vi "IndividualOperations.vi"() -> ()   [LabVIEW 2021]
panel:
  in  "Slide":cluster{dbl, dbl}(slide)={0.0, 191.73664122137404} scale=0.0..255.0
  in  "U1":dbl(slide) scale=0.0..255.0
  in  "Enum 3":T1(ring)
  in  "Enum 2":enum16{"Rojo", "Verde", "Azul", "Color"}(ring)
  out "Waveform Graph 2":dbl[][](graph)
  out "Waveform Graph":dbl[][](graph)
  out "XY Graph":cluster{i32[], dbl[]}(graph)
  out "new picture":picture
  in  "Path":path
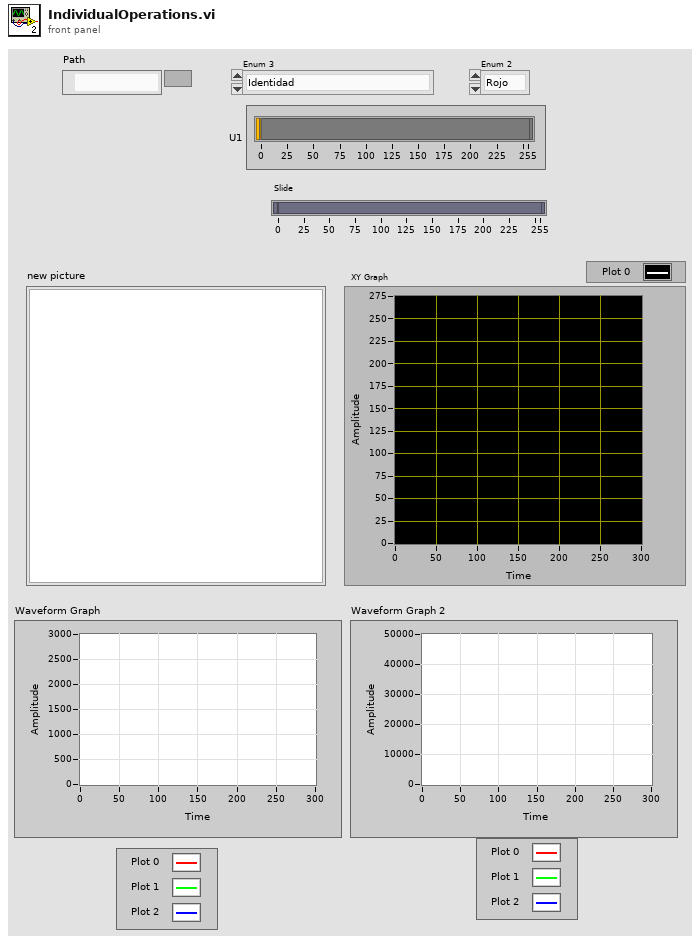
[diagram p1: front panel]
types:
  T1 = enum16{"Identidad", "Negativo", "Umbral", "Umbral Binario Por Intervalo", "Umbral Binario Por Intervalo Invertido", "Umbral Escala de Grises", "Extensión", "Reducción de nivel de grises"}
  T2 = typedef "imagedata.ctl" = cluster{"image type":i32, "image depth":i32, "image":u8[], "mask":u8[], "colors":u32[], "Rectangle":cluster{"left":i16, "top":i16, "right":i16, "bottom":i16}}
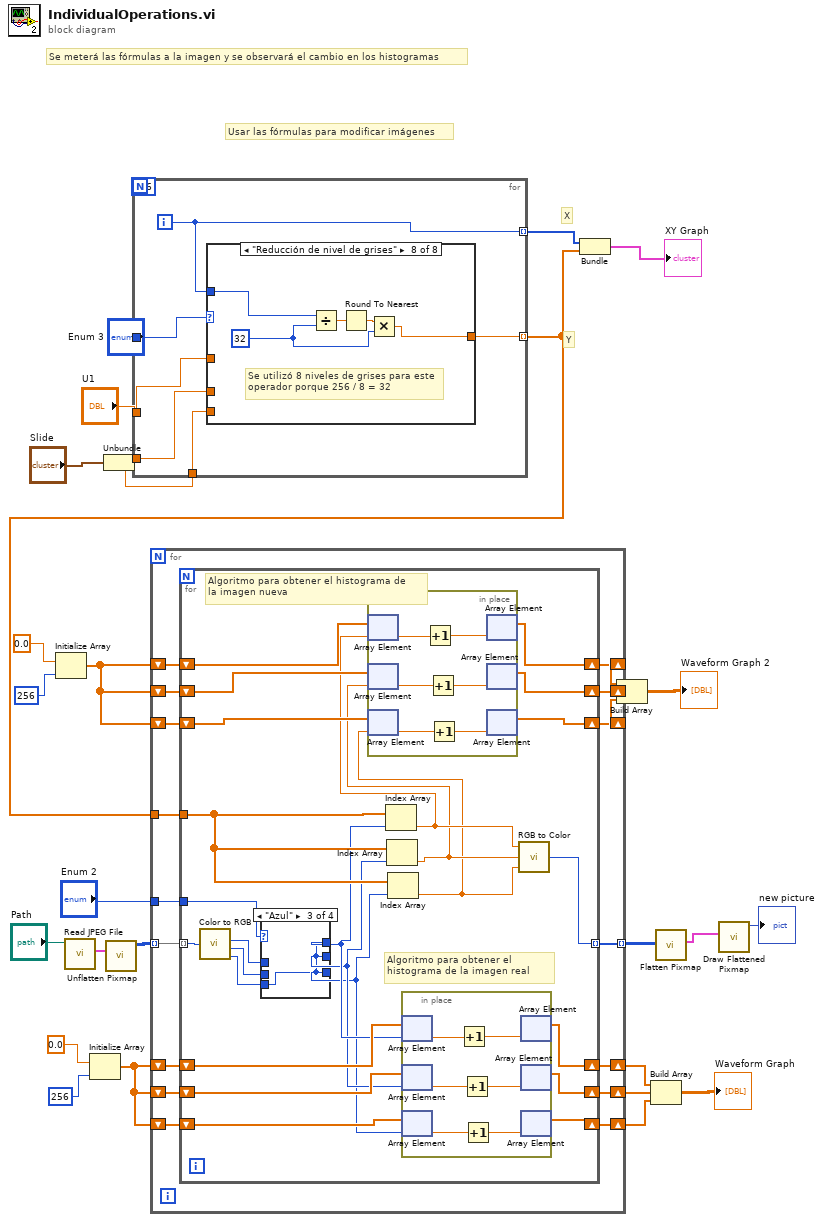
[diagram p0: block diagram]
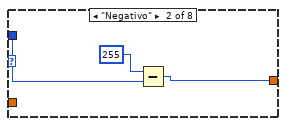
[diagram p3: hidden frame]
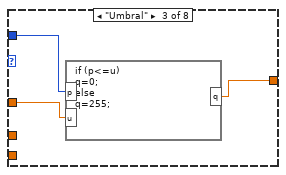
[diagram p4: hidden frame]
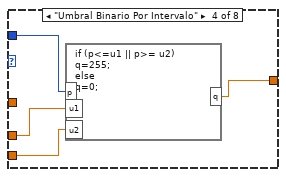
[diagram p5: hidden frame]
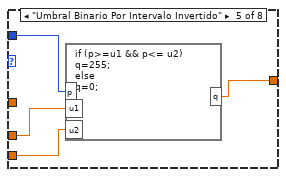
[diagram p6: hidden frame]
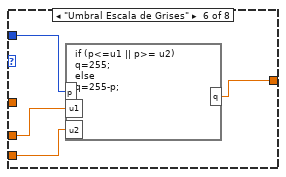
[diagram p7: hidden frame]
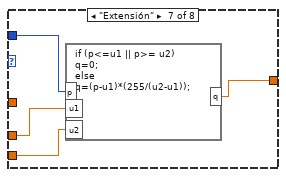
[diagram p8: hidden frame]
diagram:
  # "Usar las fórmulas para modificar imágenes"
  # "Se meterá las fórmulas a la imagen y se observará el cambio en los histogramas"
  # "Y"
  # "X"
  n1 = Initialize Array(0.0 ("element"), 256 ("dimension size")) -> (w9:dbl[])
  n2 = call <vilib>:"Read JPEG File.vi"("path to JPEG file"="Path") -> ("image data"=w29:T2)  [unwired: 8 in, 2 out]
  n3 = Initialize Array(0.0 ("element"), 256 ("dimension size")) -> (w19:dbl[])
  n4 = Unbundle("Slide") -> (w2:dbl, w1:dbl)
  n5 = call <vilib>:"Unflatten Pixmap.vi"("image data"=w29) -> ("24-bit pixmap"=w26:u32[][])  [unwired: 4 in, 6 out]
  n6 = for {
    N: 256 -> [_]
    tunnel: [w35] -> w23 mode=indexing
    tunnel: [w34] -> w14 mode=indexing
    tunnel: "Enum 3" -> [w36]
    tunnel: "U1" -> [w33]
    tunnel: w2 -> [w32]
    tunnel: w1 -> [w31]
    i -> [w35]
    n7 = case shown="\"Reducción de nivel de grises\"" w36 {
      tunnel: w35 -> [w37 w38 w43 w47 w51 w55 w59 w64]
      tunnel: [w37 w39 w41 w46 w50 w54 w58 w60] -> w34
      tunnel: w33 -> [_ _ w42 _ _ _ _ _]
      tunnel: w32 -> [_ _ _ w45 w49 w53 w57 _]
      tunnel: w31 -> [_ _ _ w44 w48 w52 w56 _]
      frame "Identidad", Default {
      }
      frame "Negativo" {
        n8 = Subtract(x=255, y=w38) -> (x-y=w39:i32)
      }
      frame "Umbral" {
        n9 = formula code="if (p<=u)\nq=0;\nelse\nq=255;"("p"=w43, "u"=w42) -> ("q"=w41:dbl)
      }
      frame "Umbral Binario Por Intervalo" {
        n10 = formula code="if (p<=u1 || p>= u2)\nq=255;\nelse\nq=0;"("p"=w47, "u1"=w45, "u2"=w44) -> ("q"=w46:dbl)
      }
      frame "Umbral Binario Por Intervalo Invertido" {
        n11 = formula code="if (p>=u1 && p<= u2)\nq=255;\nelse\nq=0;"("p"=w51, "u1"=w49, "u2"=w48) -> ("q"=w50:dbl)
      }
      frame "Umbral Escala de Grises" {
        n12 = formula code="if (p<=u1 || p>= u2)\nq=255;\nelse\nq=255-p;"("p"=w55, "u1"=w53, "u2"=w52) -> ("q"=w54:dbl)
      }
      frame "Extensión" {
        n13 = formula code="if (p<=u1 || p>= u2)\nq=0;\nelse\nq=(p-u1)*(255/(u2-u1));"("p"=w59, "u1"=w57, "u2"=w56) -> ("q"=w58:dbl)
      }
      frame "Reducción de nivel de grises" {
        w61 = 32
        # "Se utilizó 8 niveles de grises para este\noperador porque 256 / 8 = 32"
        n14 = Divide(x=w64, y=w61) -> (x/y=w63:dbl)
        n15 = Round To Nearest(number=w63) -> (nearest integer value=w62:dbl)
        n16 = Multiply(x=w62, y=w61) -> (x*y=w60:dbl)
      }
    }
  }
  n17 = for {
    tunnel: w26 -> [w80] mode=indexing
    tunnel: [w79] -> w25 mode=indexing
    shift-right: [w75] -> w18
    shift-left: w19 -> [w78]
    shift-right: [w74] -> w17
    shift-left: w19 -> [w77]
    shift-right: [w73] -> w16
    shift-left: w19 -> [w76]
    tunnel: w14 -> [w72]
    shift-right: [w69] -> w10
    shift-left: w9 -> [w66]
    shift-right: [w70] -> w11
    shift-left: w9 -> [w67]
    shift-right: [w71] -> w12
    shift-left: w9 -> [w68]
    tunnel: "Enum 2" -> [w65]
    n18 = for {
      tunnel: w80 -> [w104] mode=indexing
      tunnel: [w105] -> w79 mode=indexing
      shift-right: [w102] -> w75
      shift-left: w78 -> [w103]
      shift-right: [w99] -> w74
      shift-left: w77 -> [w101]
      shift-right: [w98] -> w73
      shift-left: w76 -> [w100]
      tunnel: w72 -> [w97]
      shift-right: [w92] -> w69
      shift-left: w66 -> [w91]
      shift-right: [w95] -> w70
      shift-left: w67 -> [w93]
      shift-right: [w96] -> w71
      shift-left: w68 -> [w94]
      tunnel: w65 -> [w87]
      # "Algoritmo para obtener el histograma de \nla imagen nueva"
      # "Algoritmo para obtener el histograma de la imagen real"
      n19 = call <vilib>:"Color to RGB.vi"("Color"=w104) -> ("R"=w81:u8, "G"=w82:u8, "B"=w83:u8)  [unwired: 1 out]
      n20 = case shown="\"Azul\"" w87 {
        tunnel: [w112 w113 w114 w117] -> w86
        tunnel: [w112 w113 w114 w116] -> w85
        tunnel: [w112 w113 w114 w115] -> w84
        tunnel: w83 -> [_ _ w114 w115]
        tunnel: w82 -> [_ w113 _ w116]
        tunnel: w81 -> [w112 _ _ w117]
        frame "Rojo", Default {
        }
        frame "Verde" {
        }
        frame "Azul" {
        }
        frame "Color" {
        }
      }
      n21 = Index Array(array=w97, index=w86) -> (element=w90:dbl)
      n22 = Index Array(array=w97, index=w85) -> (element=w89:dbl)
      n23 = Index Array(array=w97, index=w84) -> (element=w88:dbl)
      n24 = in-place {
        n25 = in-place-array #1(w91, w90) -> (w123:dbl)
        n26 = in-place-array #2(w93, w89) -> (w120:dbl)
        n27 = in-place-array #3(w94, w88) -> (w121:dbl)
        n28 = Increment(x=w123) -> (x+1=w122:dbl)
        n29 = Increment(x=w120) -> (x+1=w119:dbl)
        n30 = Increment(x=w121) -> (x+1=w118:dbl)
        n31 = in-place-array #1(w122) -> (w92:dbl[])  [unwired: 1 out]
        n32 = in-place-array #2(w119) -> (w95:dbl[])  [unwired: 1 out]
        n33 = in-place-array #3(w118) -> (w96:dbl[])  [unwired: 1 out]
      }
      n34 = in-place {
        n35 = in-place-array #4(w103, w86) -> (w111:dbl)
        n36 = in-place-array #5(w101, w85) -> (w108:dbl)
        n37 = in-place-array #6(w100, w84) -> (w109:dbl)
        n38 = Increment(x=w111) -> (x+1=w110:dbl)
        n39 = Increment(x=w108) -> (x+1=w107:dbl)
        n40 = Increment(x=w109) -> (x+1=w106:dbl)
        n41 = in-place-array #4(w110) -> (w102:dbl[])  [unwired: 1 out]
        n42 = in-place-array #5(w107) -> (w99:dbl[])  [unwired: 1 out]
        n43 = in-place-array #6(w106) -> (w98:dbl[])  [unwired: 1 out]
      }
      n44 = call <vilib>:"RGB to Color.vi"("B"=w88, "G"=w89, "R"=w90) -> ("Color"=w105:u32)
    }
  }
  n45 = Bundle(w23, w14) -> (→"XY Graph":cluster{i32[], dbl[]})  [unwired: 1 in]
  n46 = Build Array(w10, w11, w12) -> (→"Waveform Graph 2":dbl[][])
  n47 = Build Array(w18, w17, w16) -> (→"Waveform Graph":dbl[][])
  n48 = call <vilib>:"Flatten Pixmap.vi"("24-bit pixmap"=w25) -> ("image data"=w28:T2)  [unwired: 10 in]
  n49 = call <vilib>:"Draw Flattened Pixmap.vi"("image data"=w28) -> ("new picture"=→"new picture":picture)  [unwired: 8 in]
